vi "Get Class.vi"   [LabVIEW 2021, in "Multi_Bus.lvclass"]
uses:
  Multi_Bus.lvclass
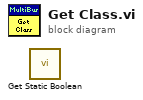
[diagram p0: block diagram]
diagram:
  n1 = call "Get Static Boolean.vi"() -> ()  [unwired: 9 in, 3 out]
